vi "MCL Trigger Read Wave Form N.vi"(7 "handle":i32, 8 "error in (no error)":errorcluster, 9 "waveform":dbl, 10 "DataPoints":u32, 11 "axis":u32) -> (0 "error out":errorcluster, 1 "waveform out":dbl, 3 "function return":i32)   [LabVIEW 2014, in "Madlib.lvlib"]
doc: "MADLIB_API int MCL_Trigger_ReadWaveFormN(unsigned int axis,unsigned int DataPoints,double *waveform, int handle);"
uses:
  <userlib>/Lambda2/lib/Madlib/Madlib.lvlib
  <userlib>/Lambda2/lib/Madlib/Madlib.dll
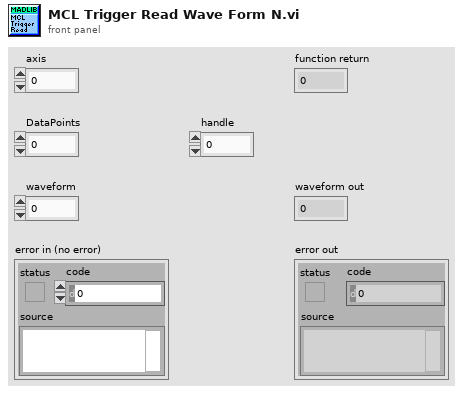
[diagram p1: front panel]
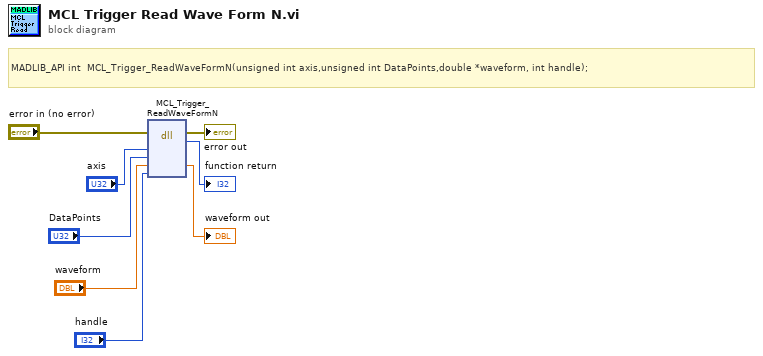
[diagram p0: block diagram]
diagram:
  # "MADLIB_API\tint\t\tMCL_Trigger_ReadWaveFormN(unsigned int axis,unsigned int DataPoints,double *waveform, int handle);"
  n1 = dll-call lib="C:/Program Files (x86)/National Instruments/LabVIEW 2014/user.lib/Lambda2/lib/Madlib/Madlib.*" fn="MCL_Trigger_ReadWaveFormN"(error in="error in (no error)", "axis"="axis", "DataPoints"="DataPoints", "waveform"="waveform", "handle"="handle") -> (error out=→"error out":errorcluster, →"function return":i32, "waveform"=→"waveform out":dbl)  [unwired: 5 in, 1 out]
